vi "Initialize Server State.vi"(8 "error in (no error)":errorcluster, 10 "Initial State":T1, 11 "gRPC Server in":refnum<class "Query Server.lvclass">) -> (0 "error out":errorcluster, 3 "gRPC Server out":refnum<class "Query Server.lvclass">)   [LabVIEW 2016, in "Query Server.lvlib" / "Query Server.lvclass"]
uses:
  Query Server.lvclass
  typeDefs/Server State Data.ctl
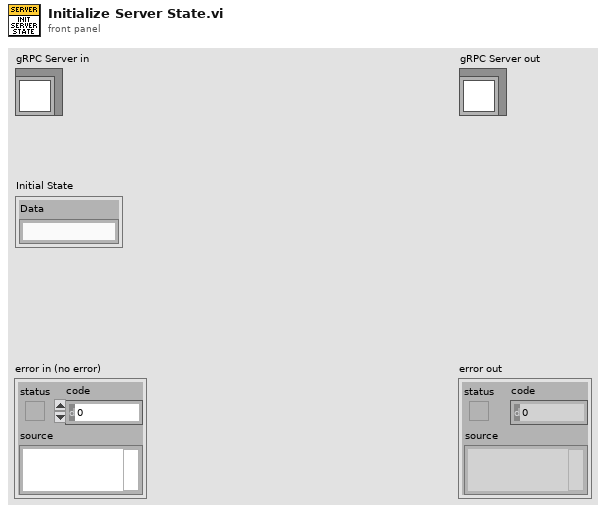
[diagram p1: front panel]
types:
  T1 = typedef "Query Server.lvlib/Query Server.lvclass/Server State Data.ctl" = cluster{"Data":string}
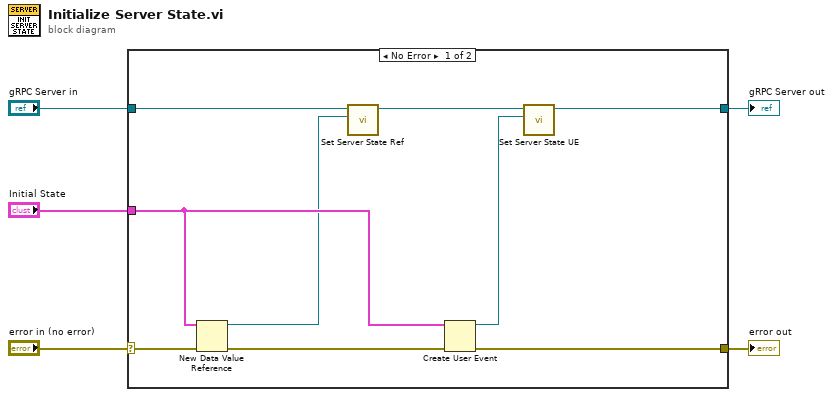
[diagram p0: block diagram]
diagram:
  n1 = case shown="No Error" "error in (no error)" {
    selector: "error in (no error)" -> [w13 w16]
    tunnel: [w12 w16] -> w4
    tunnel: [w7 w15] -> w2
    tunnel: "gRPC Server in" -> [w10 w15]
    tunnel: "Initial State" -> [w11 _]
    frame No Error {
      n2 = New Data Value Reference(data value=w11, error in=w13) -> (data value reference=w9:refnum<data-value>, error out=w14:errorcluster)
      n3 = call "Set Server State Ref.vi"("Server Internal State Ref"=w9, "Template Server in"=w10) -> ("Template Server out"=w8:refnum<class "Query Server.lvclass">)  [unwired: 9 in]
      n4 = Create User Event(user event datatype=w11, error in=w14) -> (user event=w6:refnum<user-event>, error out=w12:errorcluster)
      n5 = call "Set Server State UE.vi"("Server State UE"=w6, "Template Server in"=w8) -> ("Template Server out"=w7:refnum<class "Query Server.lvclass">)  [unwired: 9 in]
    }
    frame Error {
    }
  }
  "error out" <- w4
  "gRPC Server out" <- w2
